vi "Initialize Hardware References.vi"(8 "error in":errorcluster, 11 "Hardware Resources in":T1={"Data source"=enum."Serial port", "Connection info"={"VISA resource name"="COM 1", "Baud rate"=9600, "data bits"=8, "stop bits"=0, "parity (0:none)"=enum."None", "flow control (0:none)"=0, "timeout (10sec)"=10000, "termination char\n(0xA = '\\n' = LF) "=10, "Enable Termination\nChar (T)"=TRUE}, "Protocol info"={"Temination char"=255, "Escape char"=254}, "Internet server"={"Web page telemetry"="", "Web page gps"=""}, "Data format"=enum."IDRA data"} {"Connection info"."flow control (0:none)" items=["None", "XON/XOFF", "RTS/CTS", "XON/XOFF & RTS/CTS", "DTR/DSR", "XON/XOFF & DTR/DSR"]}) -> (0 "error out":errorcluster, 3 "Hardware Resources out":T1={"Data source"=enum."Serial port", "Connection info"={"VISA resource name"="COM 1", "Baud rate"=9600, "data bits"=8, "stop bits"=0, "parity (0:none)"=enum."None", "flow control (0:none)"=0, "timeout (10sec)"=10000, "termination char\n(0xA = '\\n' = LF) "=10, "Enable Termination\nChar (T)"=TRUE}, "Protocol info"={"Temination char"=255, "Escape char"=254}, "Internet server"={"Web page telemetry"="", "Web page gps"=""}, "Data format"=enum."IDRA data"} {"Connection info"."flow control (0:none)" items=["None", "XON/XOFF", "RTS/CTS", "XON/XOFF & RTS/CTS", "DTR/DSR", "XON/XOFF & DTR/DSR"]})   [LabVIEW 2015, in "Acquisition.lvlib"]
doc: "Initialize the hardware references."
uses:
  Acquisition.lvlib
  Hardware Configuration.ctl
  <vilib>/Instr/_visa.llb/VISA Configure Serial Port (Instr).vi
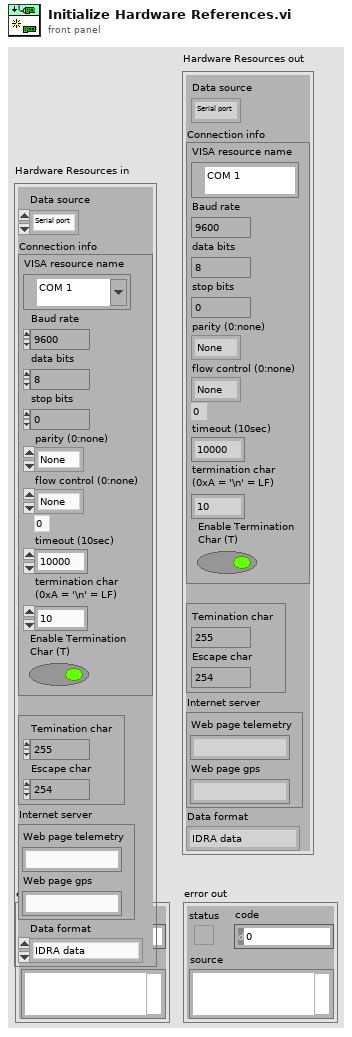
[diagram p1: front panel]
types:
  T1 = typedef "Acquisition.lvlib/Hardware Configuration.ctl" = cluster{"Data source":enum16{"Serial port", "Simulated data", "Web page JSON"}, "Connection info":cluster{"VISA resource name":refnum<visa-resource-name>, "Baud rate":u32, "data bits":u16, "stop bits":u16, "parity (0:none)":enum16{"None", "Odd", "Even", "Mark", "Space"}, "flow control (0:none)":u16, "timeout (10sec)":u32, "termination char\n(0xA = '\\n' = LF) ":u8, "Enable Termination\nChar (T)":bool}, "Protocol info":cluster{"Temination char":u8, "Escape char":u8}, "Internet server":cluster{"Web page telemetry":string, "Web page gps":string}, "Data format":enum16{"IDRA data", "XAM data"}}
  T2 = enum16{"Serial port", "Simulated data", "Web page JSON"}
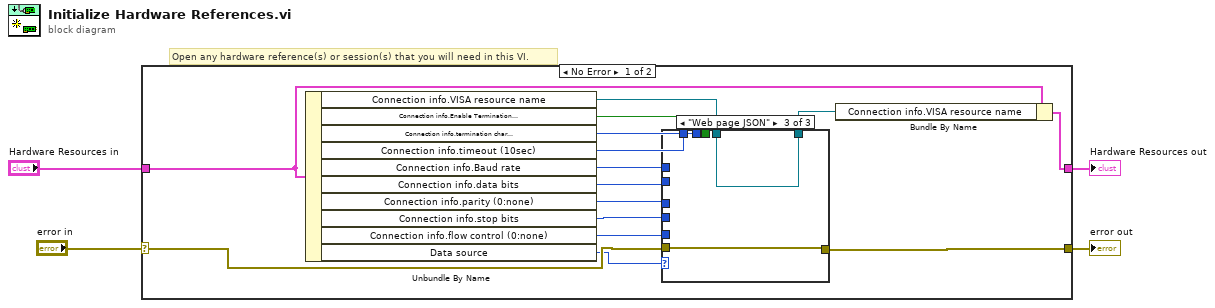
[diagram p0: block diagram]
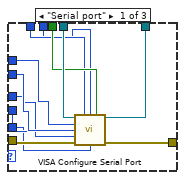
[diagram p2: hidden frame]
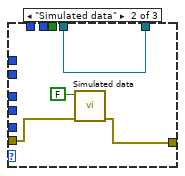
[diagram p3: hidden frame]
diagram:
  # "Open any hardware reference(s) or session(s) that you will need in this VI."
  n1 = case shown="No Error" "error in" {
    selector: "error in" -> [w17 w38]
    tunnel: [w16 w38] -> w3
    tunnel: "Hardware Resources in" -> [w18 w39]
    tunnel: [w19 w39] -> w1
    frame No Error {
      n2 = Unbundle By Name(w18) -> ("Connection info.VISA resource name"=w14:refnum<visa-resource-name>, "Connection info.Enable Termination\nChar (T)"=w12:bool, "Connection info.termination char\n(0xA = '\\n' = LF)"=w6:u8, "Connection info.timeout (10sec)"=w11:u32, "Connection info.Baud rate"=w13:u32, "Connection info.data bits"=w10:u16, "Connection info.parity (0:none)"=w9:enum16{"None", "Odd", "Even", "Mark", "Space"}, "Connection info.stop bits"=w8:u16, "Connection info.flow control (0:none)"=w7:u16, "Data source"=w5:T2)
      n3 = case shown="\"Web page JSON\"" w5 {
        tunnel: w17 -> [w31 w34 w36]
        tunnel: [w30 w33 w36] -> w16
        tunnel: [w29 w35 w37] -> w15
        tunnel: w14 -> [w28 w35 w37]
        tunnel: w13 -> [w27 _ _]
        tunnel: w12 -> [w26 _ _]
        tunnel: w11 -> [w25 _ _]
        tunnel: w10 -> [w24 _ _]
        tunnel: w9 -> [w23 _ _]
        tunnel: w8 -> [w22 _ _]
        tunnel: w7 -> [w21 _ _]
        tunnel: w6 -> [w20 _ _]
        frame "Serial port" {
          n4 = call-poly "VISA Configure Serial Port"("VISA resource name"=w28, "timeout (10sec)"=w25, "termination char\n(0xA = '\\n' = LF)"=w20, "Enable Termination\nChar (T)"=w26, "baud rate (9600)"=w27, "data bits (8)"=w24, "parity (0:none)"=w23, "error in (no error)"=w31, "stop bits (10: 1 bit)"=w22, "flow control (0:none)"=w21) -> ("VISA resource name out"=w29:refnum<visa-resource-name>, "error out"=w30:errorcluster)  [unwired: 4 in]
        }
        frame "Simulated data" {
          n5 = call "Simulated data.vi"("error in"=w34, "run/reset"=FALSE) -> ("error out"=w33:errorcluster)  [unwired: 8 in, 1 out]
        }
        frame "Web page JSON" {
        }
      }
      n6 = Bundle By Name(cluster=w18, "Connection info.VISA resource name"=w15) -> (w19:T1)
    }
    frame Error {
    }
  }
  "Hardware Resources out" <- w1
  "error out" <- w3
